vi "LogfileReader.vi"(8 "error in (no error)":errorcluster, 11 "Positions file":path) -> (0 "error out":errorcluster, 1 "Focus":dbl[](array[numeric]), 2 "Y":dbl[](array[numeric]), 3 "X":dbl[](array[numeric]), 5 "Time":dbl[](array[numeric]))   [LabVIEW 2012]
uses:
  <vilib>/Utility/file.llb/Read From Spreadsheet File (string).vi
panel:
  out "Focus vs Time":cluster{dbl, dbl}[](graph)
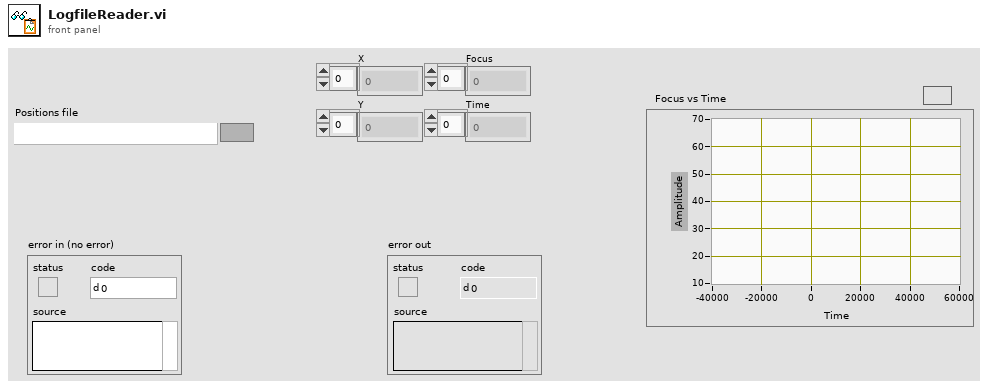
[diagram p1: front panel]
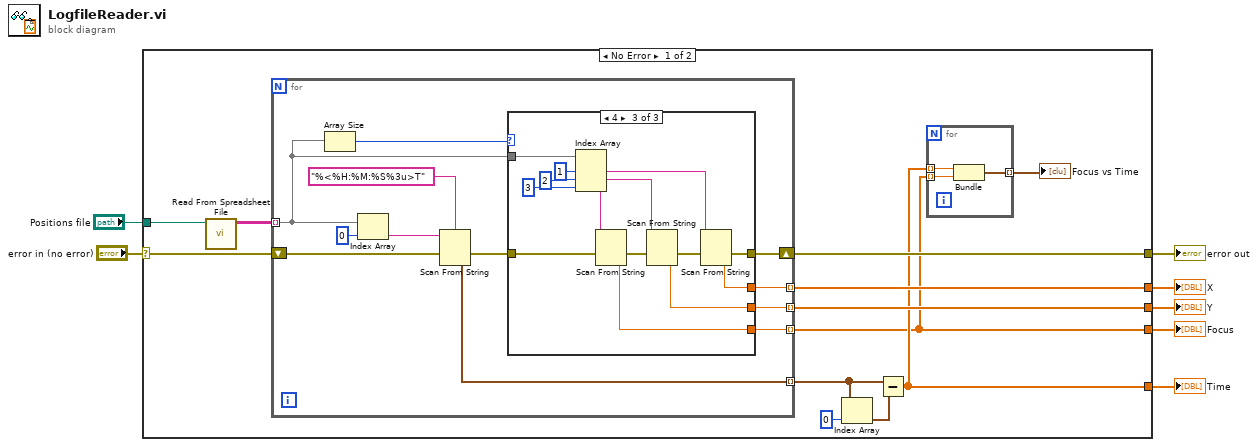
[diagram p0: block diagram]
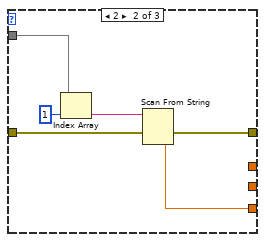
[diagram p3: hidden frame]
diagram:
  n1 = case shown="No Error" "error in (no error)" {
    selector: "error in (no error)" -> [w18 w56]
    tunnel: "Positions file" -> [w16 _]
    tunnel: [w17 w56] -> w5
    tunnel: [w10 _] -> w1
    tunnel: [w9 _] -> w2
    tunnel: [w12 _] -> w4
    tunnel: [w11 _] -> w3
    frame No Error {
      n2 = call-poly <vilib>:"Read From Spreadsheet File.vi"("file path (dialog if empty)"=w16) -> ("all rows"=w19:string[][])  [unwired: 6 in, 4 out]
      n3 = for {
        tunnel: w19 -> [w26] mode=indexing
        tunnel: [w31] -> w13 mode=indexing
        shift-right: [w27] -> w17
        shift-left: w18 -> [w30]
        tunnel: [w25] -> w9 mode=indexing
        tunnel: [w24] -> w12 mode=indexing
        tunnel: [w23] -> w11 mode=indexing
        n4 = Array Size(array=w26) -> (size(s)=w28:i32)
        n5 = Index Array(array=w26, index=0) -> (element=w33:string)
        n6 = Scan From String(format string="%<%H:%M:%S%3u>T", input string=w33, error in=w30) -> (error out=w29:errorcluster, output 1=w31:timestamp)  [unwired: 2 in, 2 out]
        n7 = case shown="4" w28 {
          tunnel: w29 -> [w35 w39 w54]
          tunnel: [w35 w37 w46] -> w27
          tunnel: w26 -> [_ w38 w53]
          tunnel: [_ w36 w52] -> w25
          tunnel: [_ _ w43] -> w24
          tunnel: [_ _ w42] -> w23
          frame 0, Default {
          }
          frame 2 {
            n8 = Index Array(array=w38, index=1) -> (element=w40:string)
            n9 = Scan From String(input string=w40, error in=w39) -> (error out=w37:errorcluster, output 1=w36:dbl)  [unwired: 3 in, 2 out]
          }
          frame 4 {
            n10 = Index Array(array=w53, index #1=1 ("index"), index #2=2 ("index"), index #3=3 ("index")) -> (element #1=w44:string, element #2=w45:string, element #3=w49:string)
            n11 = Scan From String(input string=w49, error in=w54) -> (error out=w47:errorcluster, output 1=w52:dbl)  [unwired: 3 in, 2 out]
            n12 = Scan From String(input string=w45, error in=w47) -> (error out=w48:errorcluster, output 1=w43:dbl)  [unwired: 3 in, 2 out]
            n13 = Scan From String(input string=w44, error in=w48) -> (error out=w46:errorcluster, output 1=w42:dbl)  [unwired: 3 in, 2 out]
          }
        }
      }
      n14 = Index Array(array=w13, index=0) -> (element=w14:timestamp)
      n15 = Subtract(x=w13, y=w14) -> (x-y=w10:dbl[])
      n16 = for {
        tunnel: w10 -> [w21] mode=indexing
        tunnel: w9 -> [w22] mode=indexing
        tunnel: [w20] -> w8 mode=indexing
        n17 = Bundle(w21, w22) -> (w20:cluster{dbl, dbl})  [unwired: 1 in]
      }
      "Focus vs Time" <- w8
    }
    frame Error {
    }
  }
  "error out" <- w5
  "X" <- w3
  "Y" <- w4
  "Focus" <- w2
  "Time" <- w1
